vi "Check if SV exist (import).vi"(7 "Check if SV Exists?":bool, 8 "error in (no error)":errorcluster, 11 "Channels in":refnum<class "Channel.lvclass">[](array[class])) -> (0 "error out":errorcluster, 2 "Missing Variables":string[](array[string]), 3 "Channels in 2":refnum<class "Channel.lvclass">[](array[class]))   [LabVIEW 2020, in "Shared Variables CD 2.0 Configuration.lvlib"]
uses:
  Shared Variables CD 2.0 Configuration.lvlib
  Public/Documents/National Instruments/NI VeriStand 2020/Custom Devices/Shared Variables CD 2.0/Data/Channel.lvlibp/Channel.lvclass
  Shared/SV Global.vi
  <vilib>/ErrorRing/Error Ring.xnode
  <resource>/objmgr/ni.var.rc
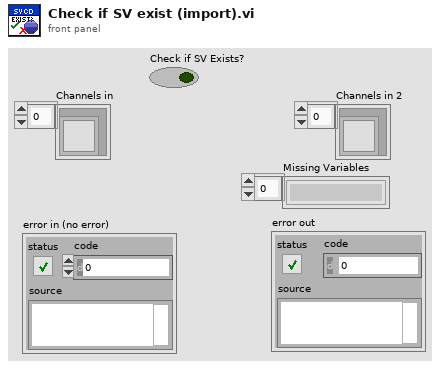
[diagram p1: front panel]
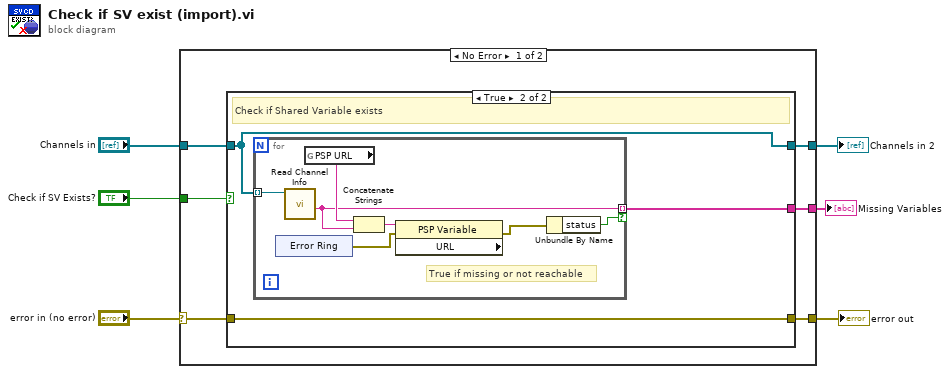
[diagram p0: block diagram]
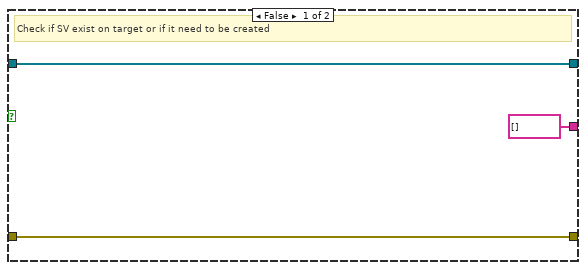
[diagram p2: hidden frame]
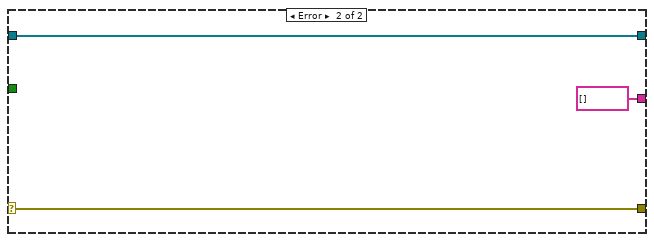
[diagram p3: hidden frame]
diagram:
  n1 = case shown="No Error" "error in (no error)" {
    selector: "error in (no error)" -> [w8 w29]
    tunnel: "Channels in" -> [w12 w28]
    tunnel: "Check if SV Exists?" -> [w11 _]
    tunnel: [w10 w29] -> w4
    tunnel: [w9 w28] -> w3
    tunnel: [w7 string[] []] -> w1
    frame No Error {
      n2 = case shown="True" w11 {
        tunnel: w8 -> [w15 w16]
        tunnel: w12 -> [w14 w18]
        tunnel: [w15 w16] -> w10
        tunnel: [w14 w18] -> w9
        tunnel: [string[] [] w17] -> w7
        frame False {
          # "Check if SV exist on target or if it need to be created"
        }
        frame True {
          # "Check if Shared Variable exists"
          n3 = for {
            tunnel: w18 -> [w25] mode=indexing
            tunnel: [w21] -> w17 mode=indexing if=w19
            # "True if missing or not reachable"
            n4 = xnode "Error Ring"() -> ("error out"=w22:errorcluster)
            n5 = call "Read Channel Info.vi"("Channel in"=w25) -> ("URL"=w21:string)  [unwired: 5 in, 5 out]
            n6 = global read "SV Global.vi" "PSP URL"() -> (w24:string)
            n7 = Concatenate Strings(w24, w21) -> (w23:string)
            n8 = property class="PSP Variable" props=["URL"](reference=w23, error in=w22) -> (error out=w20:errorcluster)  [unwired: 2 out]
            n9 = Unbundle By Name(w20) -> ("status"=w19:bool)
          }
        }
      }
    }
    frame Error {
    }
  }
  "error out" <- w4
  "Channels in 2" <- w3
  "Missing Variables" <- w1
